vi "Server Parse Commands.vi"(8 "error in":errorcluster, 11 "string":string) -> (0 "error out":errorcluster, 1 "command string":string, 2 "command data":string, 3 "command":T1=enum."Restart")   [LabVIEW 2018]
doc: "Parse server command. It will detect command ID and extract its data."
uses:
  Server Event Command.ctl
  <vilib>/Utility/error.llb/Error Cluster From Error Code.vi
  <vilib>/regexp/Match Regular Expression.xnode
  <vilib>/ErrorRing/Error Ring.xnode
  octave/infolib.lvlibp
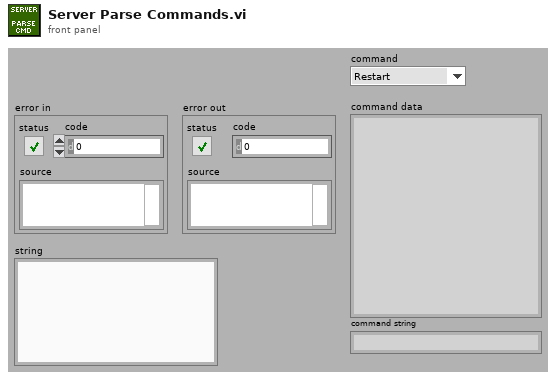
[diagram p1: front panel]
types:
  T1 = typedef "Server Event Command.ctl" = enum16{"None", "Restart", "Identify", "Set measurement", "Start", "Get status", "Get result", "Stop", "Set corrections", "Get algorithm info"}
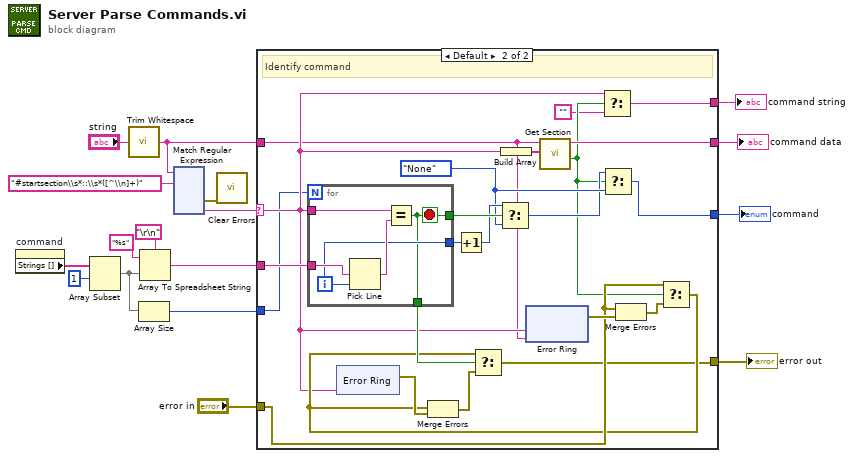
[diagram p0: block diagram]
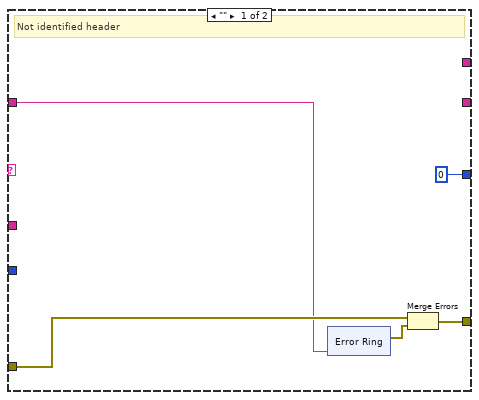
[diagram p2: hidden frame]
diagram:
  n1 = property on="command" class="Enum (strict)"() -> ("Strings []"=w7:string[])  [unwired: 2 in, 2 out]
  n2 = Array Subset(array=w7, index=1) -> (w2:string[])  [unwired: 1 in]
  n3 = call <vilib>:"Trim Whitespace.vi"("string"="string") -> ("trimmed string"=w12:string)  [unwired: 1 in]
  n4 = Array Size(array=w2) -> (size(s)=w1:i32)
  n5 = Array To Spreadsheet String(delimiter (Tab)="\r\n", array=w2, 3:"%s" ("format string")) -> (spreadsheet string=w5:string)
  n6 = xnode "Match Regular Expression"("input string"=w12, "regular expression"="#startsection\\s*::\\s*([^\\n]+)") -> ("error out"=w8:errorcluster, "submatch 1"=w15:string)  [unwired: 4 in, 4 out]
  n7 = call <vilib>:"Clear Errors.vi"("error in (no error)"=w8) -> ()  [unwired: 5 in, 2 out]
  n8 = case shown="Default" w15 {
    selector: w15 -> [_ w33]
    tunnel: w5 -> [_ w52]
    tunnel: "error in" -> [w20 w38]
    tunnel: [0 w41] -> w13
    tunnel: w12 -> [w18 w30]
    tunnel: [_ w44] -> w11
    tunnel: [w21 w36] -> w10
    tunnel: [_ w35] -> w9
    tunnel: w1 -> [_ w31]
    frame "" {
      # "Not identified header"
      n9 = xnode "Error Ring"("parameter 0"=w18) -> ("error out"=w19:errorcluster)
      n10 = Merge Errors(w20, w19) -> (w21:errorcluster)
    }
    frame Default {
      w43 = Server_Event_Command."None" ("command")
      # "Identify command"
      n11 = for {
        N: w31 -> [_]
        tunnel: w52 -> [w72]
        tunnel: w33 -> [w70]
        tunnel: [w69] -> w51
        tunnel: [w68] -> w50
        tunnel: [w68] -> w47
        i -> [w69]
        stop <- w68 stop-if-true
        n12 = Pick Line(multi-line string=w72, line index=w69) -> (output string=w71:string)  [unwired: 1 in]
        n13 = Equal?(x=w70, y=w71) -> (x = y?=w68:bool)
      }
      n14 = xnode "Error Ring"("parameter 0"=w33) -> ("error out"=w49:errorcluster)
      n15 = Increment(x=w51) -> (x+1=w46:i32)
      n16 = Select(t=w46, s=w47, f=w43) -> (s? t:f=w42:i32)
      n17 = Build Array(w33) -> (w45:string[])
      n18 = xnode "Error Ring"("parameter 0"=w33, "parameter 1"=w30) -> ("error out"=w39:errorcluster)
      n19 = call "Get Section.vi"("sections"=w45, "info data"=w30) -> ("exist"=w34:bool, "section part"=w44:string)  [unwired: 8 in]
      n20 = Select(t=w33, s=w34, f="") -> (s? t:f=w35:string)
      n21 = Select(t=w42, s=w34, f=w43) -> (s? t:f=w41:i32)
      n22 = Merge Errors(w38, w39) -> (w40:errorcluster)
      n23 = Select(t=w38, s=w34, f=w40) -> (s? t:f=w37:errorcluster)
      n24 = Merge Errors(w37, w49) -> (w48:errorcluster)
      n25 = Select(t=w37, s=w50, f=w48) -> (s? t:f=w36:errorcluster)
    }
  }
  "error out" <- w10
  "command" <- w13
  "command data" <- w11
  "command string" <- w9
